vi "StahlPS_USB.SetVoltage.vi"(0 "i ref in":refnum<vi>, 2 "value":dbl, 5 "error in (no error)":errorcluster, 7 "channelIndex":i32) -> (14 "i ref out":refnum<vi>, 19 "error out (no error)":errorcluster)   [LabVIEW 2014, in "StahlPS_USB.lvlib"]
doc: "This VI calculates the right current from the DB values, saves the actual set current to the I-Attribute and set´s the Set Current-Service."
uses:
  StahlPS_USB.lvlib
  CSCore/CSSystem/CoreDefs/CoreDefs.error_type.ctl
  CSCore/CSSystem/CoreDefs/CoreDefs.error_severity.ctl
  CSCore/CSApplicationBaseClasses/PSChannelBase/PSChannelBase.directionType.ctl
  CSCore/CSApplicationBaseClasses/PSChannelBase/PSChannelBase.serviceType.ctl
  CSlibraries/UtilityLib/UtilityLib.valueStatus.ctl
  CSCore/CSSystem/CoreLib/CoreLib.lvlib
  CSlibraries/UtilityLib/UtilityLib.lvlib
  CSCore/CSApplicationBaseClasses/PSChannelBase/PSChannelBase.lvlib
  CSinstr.lib/SE_HV_Driver/SE-HV_Driver.lvlib
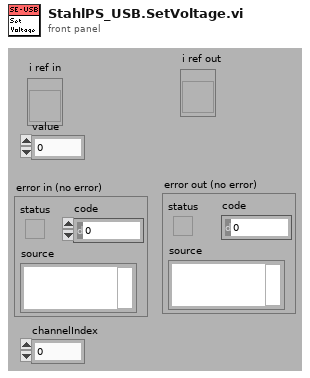
[diagram p1: front panel]
types:
  T1 = typedef "CoreDefs.error_severity.ctl" = enum16{"undefined", "information", "warning", "error", "fatal"}
  T2 = typedef "CoreDefs.error_type.ctl" = enum16{"no error", "can't load process", "can't unload process", "process does not exist", "can't install process", "can't remove process", "unknown function", "time out", "can't execute function", "duplicate queue name", "super not found", "caller queue invalid", "can't ping process", "unknown error", "VISA Error", "VISA timeout", "GPIB timeout", "GPIB error", "communication error", "data type mismatch", "can't read data from OPC server", "can't write data to OPC server", "OET error", "function not implemented", "process already exists", "invalid Shared Variable name", "error writing Shared Variable", "error reading Shared Variable", "invalid client name", "corrupt database", "unknown class", "call not authorized", "parameter out of range", "OET timeout: can't get data to modify", "invalid queue name", "requested operation incompatible with current state", "event undefined", "event disabled", "state undefined", "caller is not a friend", "EventBuilder: bad eventID", "EventBuilder: no DAQ devices", "a thread must not stop itself", "UNUSED ELEMENT4", "DiscArchiver: eventData incomplete", "DiscArchiver: eventData does not belong to run", "DiscArchiver: can't open file", "DiscArchiver: can't write to file", "DiscArchiver: available disc space low", "can't acquire semaphore", "error reading data from database", "notifier object is not existing", "can't register process", "can't unregister process", "illegal event type", "object disabled", "object already exists", "can't change state", "Instrument not found", "no connection to remote node", "invalid reference", "N/A", "UNUSED ELEMENT 1", "element not found", "illegal TCP/IP connection detected", "object does not exist", "invalid access ID", "unknown CS system", "invalid privilige", "unsupported data type", "unsupported server type", "IO server already exists", "Shared Variable already exists"}
  T3 = typedef "UtilityLib.lvlib/UtilityLib.valueStatus.ctl" = enum16{"no info available", "stand by/off", "on", "warning", "alarm/malfunction", "not implemented", "user action required", "important information", "system default", "control default", "indicator default", "button default"}
  T4 = typedef "PSChannelBase.lvlib/PSChannelBase.serviceType.ctl" = enum16{"onOff", "voltage", "current", "tripCurrent", "rampUpSpeed", "rampDownSpeed", "status"}
  T5 = typedef "PSChannelBase.lvlib/PSChannelBase.directionType.ctl" = enum16{"unknown", "update actual value", "update nominal value", "update both"}
  T6 = typedef "StahlPS_USB.lvlib/StahlPS_USB.i attribute.ctl" = cluster{"VISA resource name":refnum<visa-resource-name>, "Type":string, "MaxVoltage":dbl, "MinVoltage":dbl, "Elektrode Names":string[]}
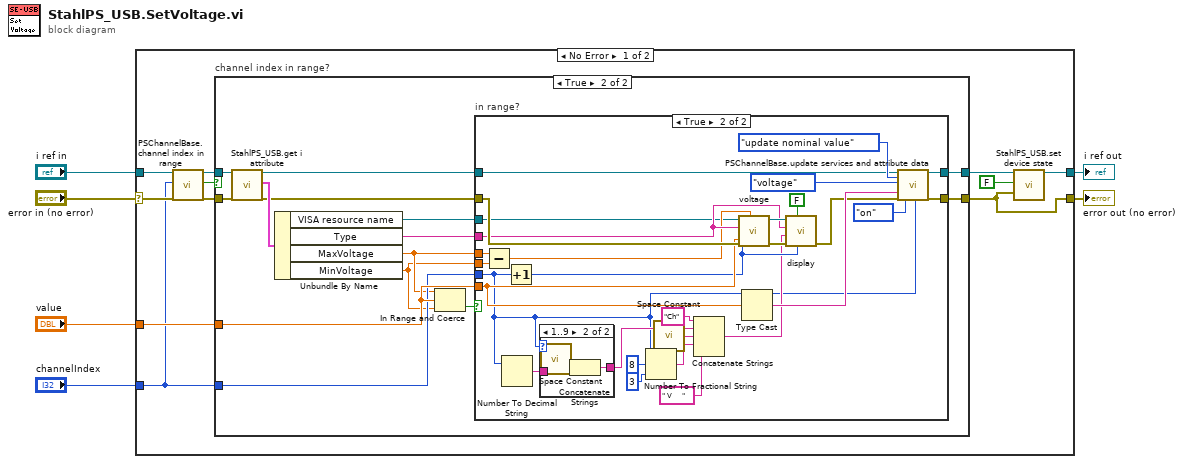
[diagram p0: block diagram]
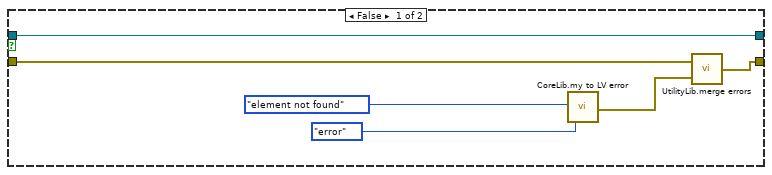
[diagram p2: hidden frame]
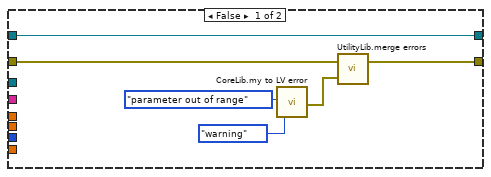
[diagram p3: hidden frame]
diagram:
  n1 = case shown="No Error" "error in (no error)" {
    selector: "error in (no error)" -> [w16 w78]
    tunnel: [w10 w78] -> w3
    tunnel: "i ref in" -> [w15 w77]
    tunnel: [w9 w77] -> w5
    tunnel: "value" -> [w17 _]
    tunnel: "channelIndex" -> [w7 _]
    frame No Error {
      n2 = call "PSChannelBase.channel index in range.vi"("i ref in"=w15, "channelIndex"=w7, "error in (no error)"=w16) -> ("i ref out"=w12:refnum<vi>, "in range"=w13:bool, "error out"=w14:errorcluster)  [unwired: 14 in]
      n3 = case "channel index in range?" shown="True" w13 {
        tunnel: w12 -> [w23 w35]
        tunnel: [w23 w34] -> w11
        tunnel: w14 -> [w20 w33]
        tunnel: [w18 w32] -> w10
        tunnel: w17 -> [_ w29]
        tunnel: w7 -> [_ w26]
        frame False {
          n4 = call "CoreLib.my to LV error.vi"("ErrorTypes"=CoreDefs.error_type."element not found", "severityLevel"=CoreDefs.error_severity."error") -> ("myErrorCluster"=w19:errorcluster)  [unwired: 16 in, 1 out]
          n5 = call "UtilityLib.merge errors.vi"("error2 (no error)"=w19, "error1 (no error)"=w20) -> ("error out"=w18:errorcluster)
        }
        frame True {
          n6 = call "StahlPS_USB.get i attribute.vi"("i ref in"=w35, "error in (no error)"=w33) -> ("i ref out"=w30:refnum<vi>, "i attribute"=w37:T6, "error out"=w31:errorcluster)  [unwired: 15 in]
          n7 = Unbundle By Name(w37) -> ("VISA resource name"=w28:refnum<visa-resource-name>, "Type"=w27:string, "MaxVoltage"=w25:dbl, "MinVoltage"=w24:dbl)
          n8 = In Range and Coerce(upper limit=w25, x=w29, lower limit=w24) -> (In Range?=w36:bool)  [unwired: 1 out]
          n9 = case "in range?" shown="True" w36 {
            tunnel: w31 -> [w41 w63]
            tunnel: [w39 w71] -> w32
            tunnel: w29 -> [_ w61]
            tunnel: w30 -> [w38 w66]
            tunnel: [w38 w72] -> w34
            tunnel: w28 -> [_ w46]
            tunnel: w27 -> [_ w62]
            tunnel: w26 -> [_ w47]
            tunnel: w25 -> [_ w60]
            tunnel: w24 -> [_ w59]
            frame False {
              n10 = call "CoreLib.my to LV error.vi"("ErrorTypes"=CoreDefs.error_type."parameter out of range", "severityLevel"=CoreDefs.error_severity."warning") -> ("myErrorCluster"=w40:errorcluster)  [unwired: 16 in, 1 out]
              n11 = call "UtilityLib.merge errors.vi"("error2 (no error)"=w40, "error1 (no error)"=w41) -> ("error out"=w39:errorcluster)
            }
            frame True {
              n12 = Subtract(x=w60, y=w59) -> (x-y=w58:dbl)
              n13 = Number To Decimal String(number=w47) -> (decimal integer string=w50:string)  [unwired: 1 in]
              n14 = Increment(x=w47) -> (x+1=w56:i32)
              n15 = case shown="1..9" w47 {
                tunnel: w50 -> [w73 w76]
                tunnel: [w73 w74] -> w49
                frame Default {
                }
                frame 1..9 {
                  n16 = call <vilib>:"Space Constant.vi"() -> ("String"=w75:string)
                  n17 = Concatenate Strings(w75, w76) -> (w74:string)
                }
              }
              n18 = Number To Fractional String(number=w47, width (-)=8, precision (6)=3) -> (F-format string=w55:string)  [unwired: 1 in]
              n19 = call <vilib>:"Space Constant.vi"() -> ("String"=w51:string)
              n20 = Concatenate Strings("Ch" ("string"), w49, w51, w55, " V     " ("string")) -> (w48:string)
              n21 = call "voltage.vi"("Voltage"=w61, "Span"=w58, "Error in"=w63, "Channel nr."=w56, "Device name"=w62, "VISA resource name in"=w46) -> ("Error out"=w65:errorcluster, "Visa resource name out"=w64:refnum<visa-resource-name>)  [unwired: 3 in, 1 out]
              n22 = Type Cast(x=w61) -> (*(type *) &x=w70:string)  [unwired: 1 in]
              n23 = call "display.vi"("Line number"=w56, "Next free line"=FALSE, "Error in"=w65, "Display String"=w48, "Device name"=w62, "VISA resource name in"=w64) -> ("Error out"=w44:errorcluster)  [unwired: 4 in, 1 out]
              n24 = call "PSChannelBase.update services and attribute data.vi"("i ref in"=w66, "direction"=PSChannelBase.directionType."update nominal value", "service"=PSChannelBase.serviceType."voltage", "value"=w70, "error in (no error)"=w44, "quality"=UtilityLib.valueStatus."on", "channelNumber"=w47) -> ("i ref out"=w72:refnum<vi>, "error out"=w71:errorcluster)  [unwired: 10 in, 1 out]
            }
          }
        }
      }
      n25 = call "StahlPS_USB.set device state.vi"("i ref in"=w11, "implicit"=FALSE, "device error"=w10) -> ("i ref out"=w9:refnum<vi>)  [unwired: 14 in, 2 out]
    }
    frame Error {
    }
  }
  "error out (no error)" <- w3
  "i ref out" <- w5
